vi "Transcriptor LabVIEW to C code Arduino Frontend.vi"(8 "error in":errorcluster, 9 "Defines":string[](array[string])=["using namespace std;"], 10 "Includes":string[](array[string])=["<ArduinoSTL.h>", "<vector>"], 11 "vi path":path) -> (0 "error out":errorcluster, 3 "transcripted code":string)   [LabVIEW 2014]
panel:
  # "Use Arduino.h just for arduino\nNO for ESP8266!"
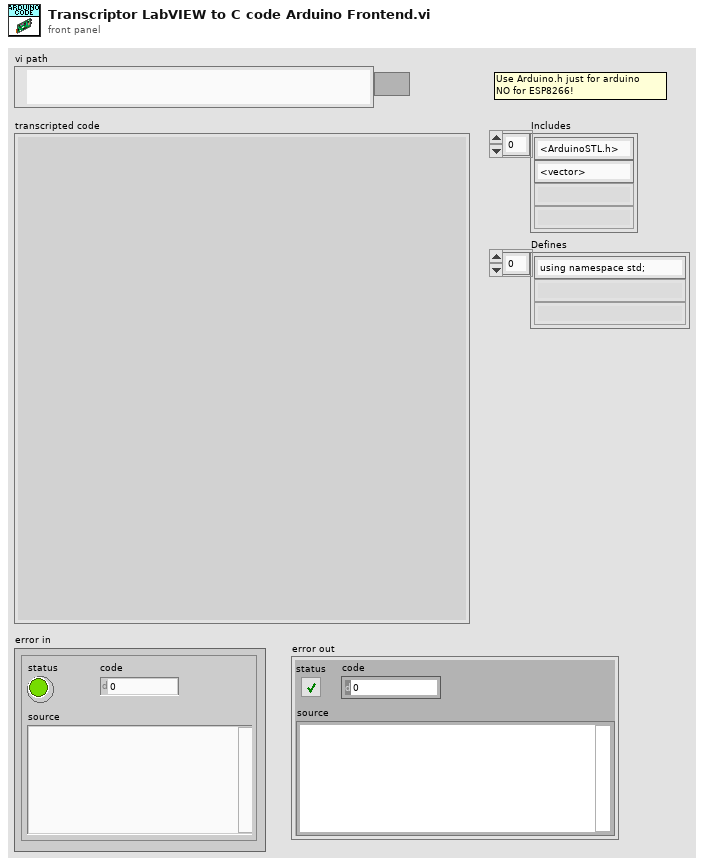
[diagram p1: front panel]
types:
  T1 = typedef "LabVIEW Universal Transcriptor Cluster.ctl" = cluster{"Defines":string[], "Includes":string[], "C code":string, "temp":string[], "temp 2":string[]}
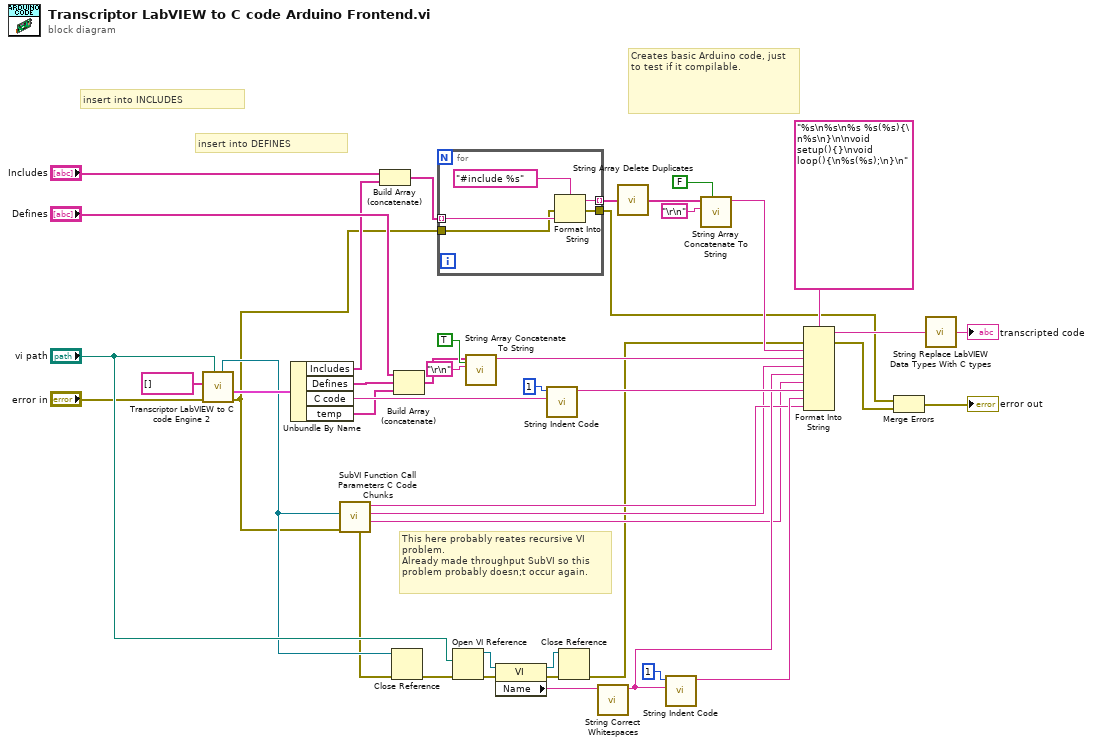
[diagram p0: block diagram]
diagram:
  # "This here probably reates recursive VI problem.\nAlready made throughput SubVI so this problem probably doesn;t occur again."
  # "insert into INCLUDES"
  # "insert into DEFINES"
  # "Creates basic Arduino code, just to test if it compilable."
  n1 = call "Transcriptor LabVIEW to C code Engine 2.vi"("VI path"="vi path", "Error In"="error in", "List Reentrant VIs"=string[] []) -> ("error out"=w3:errorcluster, "output cluster"=w44:T1, "VI ref."=w11:refnum<vi>)  [unwired: 4 in, 2 out]
  n2 = Unbundle By Name(w44) -> ("Includes"=w22:string[], "Defines"=w25:string[], "C code"=w33:string, "temp"=w13:string[])
  n3 = call "SubVI Function Call Parameters C Code Chunks.vi"("Error In"=w3, "VI Reference"=w11) -> ("SubVI func. declaration"=w17:string, "return datatype"=w18:string, "SubVI func. call in code"=w19:string, "Error Out"=w10:errorcluster)  [unwired: 4 in, 2 out]
  n4 = Build Array (concatenate)("Includes", w22) -> (w21:string[])
  n5 = Close Reference(reference=w11, error in (no error)=w10) -> (error out=w12:errorcluster)
  n6 = Build Array (concatenate)("Defines", w25, w13) -> (w24:string[])
  n7 = for {
    tunnel: w21 -> [w48] mode=indexing
    tunnel: [w47] -> w9 mode=indexing
    tunnel: w3 -> [w46]
    tunnel: [w45] -> w4
    n8 = Format Into String(format string="#include %s", error in=w46, w48) -> (resulting string=w47:string, error out=w45:errorcluster)  [unwired: 1 in]
  }
  n9 = Open VI Reference(vi path="vi path", error in (no error)=w12) -> (vi reference=w15:refnum<vi>, error out=w36:errorcluster)  [unwired: 4 in]
  n10 = call "String Array Concatenate To String.vi"("insert last delimiter?"=TRUE, "Delimiter char"="\r\n", "Array String In"=w24) -> ("String"=w41:string)  [unwired: 8 in]
  n11 = property class="VI"(reference=w15, error in=w36) -> (reference out=w16:refnum<vi>, error out=w34:errorcluster, "Name"=w35:string)
  n12 = call "String Indent Code.vi"("complete code"=w33, "actual nested level"=1) -> ("indented code"=w32:string)  [unwired: 9 in]
  n13 = Close Reference(reference=w16, error in (no error)=w34) -> (error out=w7:errorcluster)
  n14 = call "String Correct Whitespaces.vi"("String in"=w35) -> ("String out"=w29:string)  [unwired: 10 in]
  n15 = call "String Array Delete Duplicates.vi"("Array"=w9) -> ("Output array"=w8:string[])
  n16 = call "String Indent Code.vi"("complete code"=w29, "actual nested level"=1) -> ("indented code"=w28:string)  [unwired: 9 in]
  n17 = call "String Array Concatenate To String.vi"("insert last delimiter?"=FALSE, "Delimiter char"="\r\n", "Array String In"=w8) -> ("String"=w37:string)  [unwired: 8 in]
  n18 = Format Into String(format string="%s\n%s\n%s %s(%s){\n%s\n}\n\nvoid setup(){}\nvoid loop(){\n%s(%s);\n}\n", error in=w7, w37, w41, w18, w29, w17, w32, w28, w19) -> (resulting string=w27:string, error out=w5:errorcluster)  [unwired: 1 in]
  n19 = Merge Errors(w4, w5) -> (→"error out":errorcluster)
  n20 = call "String Replace LabVIEW Data Types With C types.vi"("C code"=w27) -> ("C code, replaced datatypes"=→"transcripted code":string)
